vi "face_check_subVI.vi"(9 "Lips Match":T1(array[cluster]), 10 "Nose Match":T1(array[cluster]), 11 "Eye Match":T1(array[cluster])) -> (1 "Face Rectangle":T2, 2 "Lip Position":cluster{"x":sgl, "y":sgl}, 3 "Face Found":bool)   [LabVIEW 2013]
panel:
  in  "Rectangle":T2
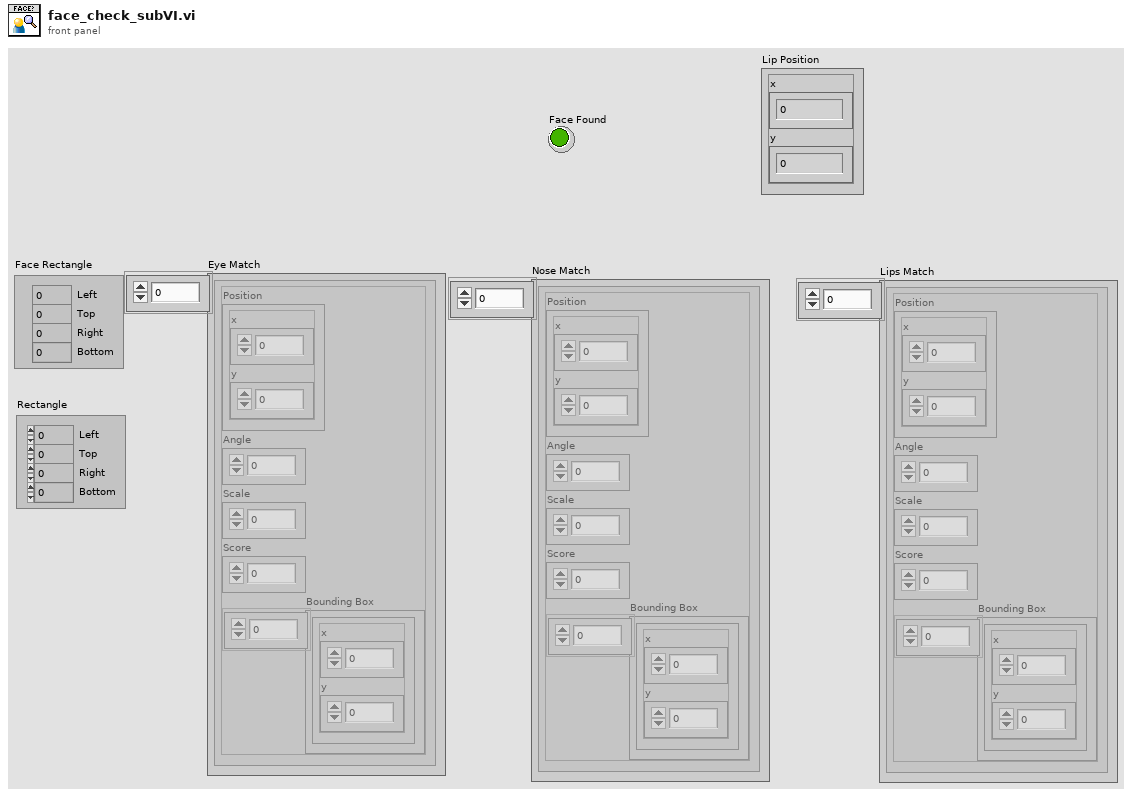
[diagram p1: front panel]
types:
  T1 = cluster{"Position":cluster{"x":sgl, "y":sgl}, "Angle":sgl, "Scale":sgl, "Score":sgl, "Bounding Box":cluster{"x":sgl, "y":sgl}[]}[]
  T2 = cluster{"Left":i32, "Top":i32, "Right":i32, "Bottom":i32}
  T3 = cluster{"Position":cluster{"x":sgl, "y":sgl}, "Angle":sgl, "Scale":sgl, "Score":sgl, "Bounding Box":cluster{"x":sgl, "y":sgl}[]}
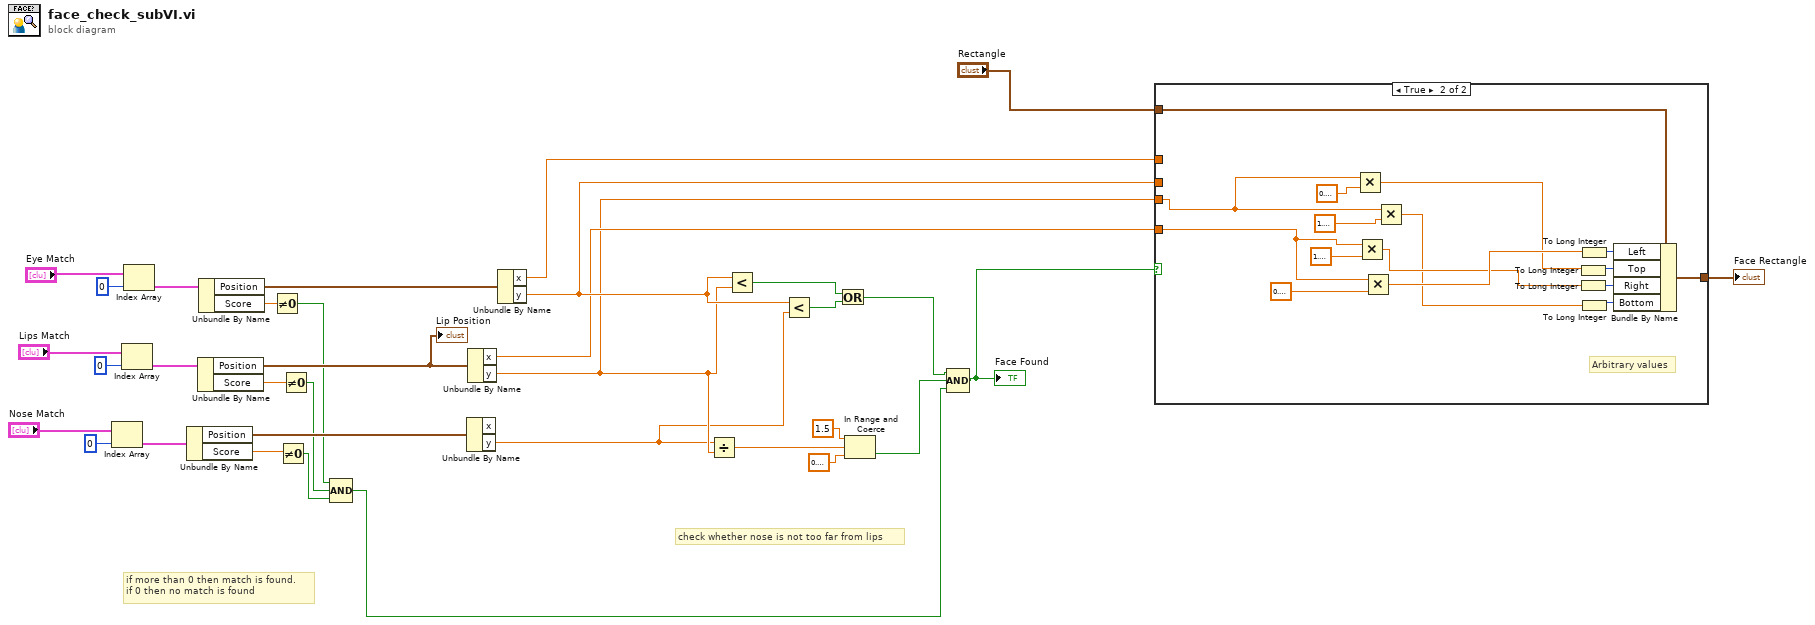
[diagram p0: block diagram]
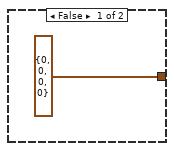
[diagram p2: hidden frame]
diagram:
  # "check whether nose is not too far from lips"
  # "if more than 0 then match is found.\nif 0 then no match is found"
  n1 = Index Array(array="Nose Match", index=0) -> (element=w16:T3)
  n2 = Index Array(array="Lips Match", index=0) -> (element=w22:T3)
  n3 = Index Array(array="Eye Match", index=0) -> (element=w23:T3)
  n4 = Unbundle By Name(w16) -> ("Position"=w15:cluster{"x":sgl, "y":sgl}, "Score"=w8:sgl)
  n5 = Unbundle By Name(w22) -> ("Position"=w19:cluster{"x":sgl, "y":sgl}, "Score"=w9:sgl)
  "Lip Position" <- w19
  n6 = Unbundle By Name(w23) -> ("Position"=w25:cluster{"x":sgl, "y":sgl}, "Score"=w10:sgl)
  n7 = Not Equal To 0?(x=w10) -> (x != 0?=w7:bool)
  n8 = Not Equal To 0?(x=w8) -> (x != 0?=w5:bool)
  n9 = Not Equal To 0?(x=w9) -> (x != 0?=w6:bool)
  n10 = Compound Arithmetic op=AND(w7, w6, w5) -> (w2:bool)
  n11 = Unbundle By Name(w15) -> ("y"=w11:sgl)  [unwired: 1 out]
  n12 = Unbundle By Name(w19) -> ("x"=w13:sgl, "y"=w12:sgl)
  n13 = Unbundle By Name(w25) -> ("x"=w29:sgl, "y"=w14:sgl)
  n14 = Divide(x=w11, y=w12) -> (x/y=w32:sgl)
  n15 = Less?(x=w14, y=w12) -> (x < y?=w33:bool)
  n16 = Less?(x=w14, y=w11) -> (x < y?=w34:bool)
  n17 = Or(x=w33, y=w34) -> (x .or. y?=w4:bool)
  n18 = In Range and Coerce(upper limit=sgl 1.5, x=w32, lower limit=sgl 0.8) -> (In Range?=w3:bool)  [unwired: 1 out]
  n19 = Compound Arithmetic op=AND(w4, w3, w2) -> (w1:bool)
  "Face Found" <- w1
  n20 = case shown="True" w1 {
    tunnel: w14 -> [_ _]
    tunnel: w12 -> [_ w48]
    tunnel: w29 -> [_ _]
    tunnel: "Rectangle" -> [_ w51]
    tunnel: [T2 {"Left"=0, "Top"=0, "Right"=0, "Bottom"=0} ("Rectangle") w50] -> w27
    tunnel: w13 -> [_ w49]
    frame False {
    }
    frame True {
      # "Arbitrary values"
      n21 = Multiply(x=w48, y=sgl 0.2) -> (x*y=w41:sgl)
      n22 = Multiply(x=w49, y=sgl 1.2) -> (x*y=w42:sgl)
      n23 = Multiply(x=w49, y=sgl 0.7) -> (x*y=w43:sgl)
      n24 = Multiply(x=w48, y=sgl 1.1) -> (x*y=w40:sgl)
      n25 = To Long Integer(number=w41) -> (32bit integer=w45:i32)
      n26 = To Long Integer(number=w42) -> (32bit integer=w46:i32)
      n27 = To Long Integer(number=w43) -> (32bit integer=w44:i32)
      n28 = To Long Integer(number=w40) -> (32bit integer=w47:i32)
      n29 = Bundle By Name(cluster=w51, "Left"=w44, "Top"=w45, "Right"=w46, "Bottom"=w47) -> (w50:T2)
    }
  }
  "Face Rectangle" <- w27
